vi "Example DUT_clinet.vi"(8 "error in":errorcluster) -> (0 "error out":errorcluster)   [LabVIEW 2012]
uses:
  TypeDef/Send Command Message.ctl
panel:
  in  "Send Command":T1
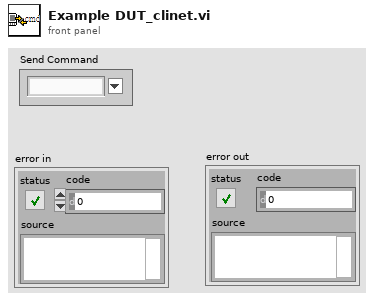
[diagram p1: front panel]
types:
  T1 = typedef "Send Command Message.ctl" = string
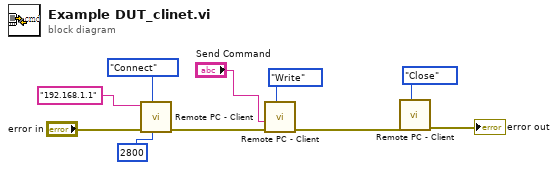
[diagram p0: block diagram]
diagram:
  n1 = call "Remote PC - Client.vi"("Remote Sever Port (2800)"=u16 2800 ("port"), "Flow Contorl"=enum16{"Connect", "Read", "Write", "Close"}."Connect" ("TCP ctrl"), "error in"="error in", "IP Address"="192.168.1.1" ("address")) -> ("error out"=w7:errorcluster)  [unwired: 6 in, 1 out]
  n2 = call "Remote PC - Client.vi"("Flow Contorl"=enum16{"Connect", "Read", "Write", "Close"}."Write" ("TCP ctrl"), "error in"=w7, "Send Command"="Send Command") -> ("error out"=w6:errorcluster)  [unwired: 7 in, 1 out]
  n3 = call "Remote PC - Client.vi"("Flow Contorl"=enum16{"Connect", "Read", "Write", "Close"}."Close" ("TCP ctrl"), "error in"=w6) -> ("error out"=→"error out":errorcluster)  [unwired: 8 in, 1 out]
